vi "Write Control.vi"(6 "Data":u8[](array[numeric]), 8 "Error In":errorcluster, 9 "Device State":u32 format="%.0x", 10 "ADS State":T4, 11 "AMS Connection In":T1) -> (0 "Error Out":errorcluster, 2 "ADS Error":T3 items=["NoError"=0, "InternalError"=1, "NoRTime"=2, "LockedMemoryError"=3, "MailBoxError"=4, "WrongHMsg"=5, "TargetPortNotFound"=6, "TargetMachineNotFound"=7, "UnknownCommandID"=8, "BadTaskID"=9, "NoIO"=10, "UnknownAmsCommand"=11, "Win32Error"=12, "PortNotConnected"=13, "InvalidAmsLength"=14, "InvalidAmsNetID"=15, "AmsSyncAmsError"=22, "AmsSyncNoIndexMap"=23, "InvalidAmsPort"=24, "NoMemory"=25, "TCPSendError"=26, "HostUnreachable"=27, "NoLockedMemory"=1280, "MailboxFull"=1282, "DeviceError"=1792, "DeviceServiceNotSupported"=1793, "DeviceInvalidGroup"=1794, "DeviceInvalidOffset"=1795, "DeviceInvalidAccess"=1796, "DeviceInvalidSize"=1797, "DeviceInvalidData"=1798, "DeviceNotReady"=1799, "DeviceBusy"=1800, "DeviceInvalidContext"=1801, "DeviceNoMemory"=1802, "DeviceInvalidParam"=1803, "DeviceNotFound"=1804, "DeviceSyntaxError"=1805, "DeviceIncompatible"=1806, "DeviceExists"=1807, "DeviceSymboldNotFound"=1808, "DeviceSymbolVersionInvalid"=1809, "DeviceInvalidState"=1810, "DeviceTransModeNotSupported"=1811, "DeviceNotifyHandleInvalid"=1812, "DeviceClientUnknown"=1813, "DeviceNoMoreHandles"=1814, "DeviceInvalidWatchsize"=1815, "DeviceNotInitialized"=1816, "DeviceTimeOut"=1817, "DeviceNoInterface"=1818, "DeviceInvalidInterface"=1819, "DeviceInvalidCLSID"=1820, "DeviceInvalidObjectID"=1821, "ClientError"=1856, "ClientInvalidParameter"=1857, "ClientListEmpty"=1858, "ClientVariableInUse"=1859, "ClientDuplicateInvokeID"=1860, "ClientSyncTimeOut"=1861, "ClientW32OR"=1862, "ClientTimeoutInvalid"=1863, "ClientPortNotOpen"=1864, "ClientNoAmsAddr"=1865, "ClientSyncInternal"=1872, "ClientAddHash"=1873, "ClientRemoveHash"=1874, "ClientNoMoreSymbols"=1875, "ClientSyncResInvalid"=1876, "ClientSyncPortLocked"=1877, "ClientQueueFull"=1878], 3 "AMS Connection Out":T1)   [LabVIEW 2016, in "TwinCAT ADS.lvlib"]
uses:
  TwinCAT ADS.lvlib
  Low Level/TypeDefs/ADS States.ctl
  Low Level/TypeDefs/ADS Error.ctl
  Low Level/TypeDefs/AMS Connection.ctl
  Low Level/TypeDefs/AMS.ctl
  Low Level/TypeDefs/Command Id.ctl
  Low Level/TypeDefs/State Flag.ctl
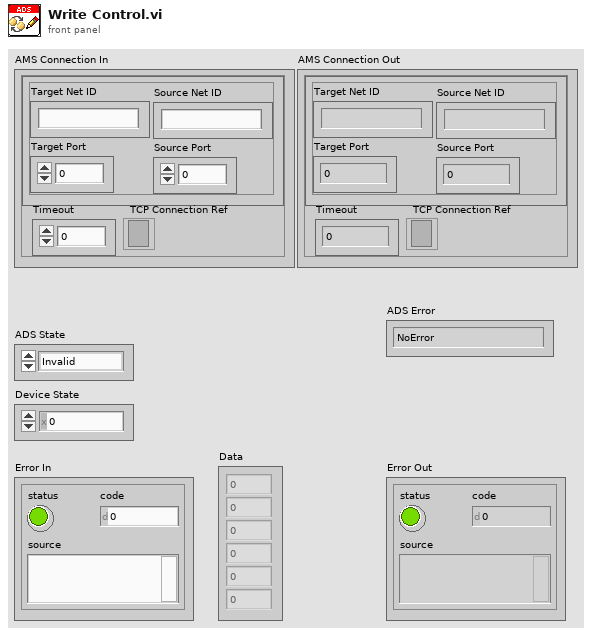
[diagram p1: front panel]
types:
  T1 = typedef "TwinCAT ADS.lvlib/AMS Connection.ctl" = cluster{"AMS":T2, "Timeout":i32, "TCP Connection Ref":refnum<k5>}
  T2 = typedef "TwinCAT ADS.lvlib/AMS.ctl" = cluster{"Target Net ID":string, "Target Port":u16, "Source Net ID":string, "Source Port":u16}
  T3 = typedef "TwinCAT ADS.lvlib/ADS Error.ctl" = i32
  T4 = typedef "TwinCAT ADS.lvlib/ADS States.ctl" = enum16{"Invalid", "Idle", "Reset", "Init", "Start", "Run", "Stop", "SaveCfg", "LoadCfg", "PowerFailure", "PowerGood", "Error", "Shutdown", "Suspend", "Resume", "Config", "Reconfig"}
  T5 = enum16{"Standard", "Buffered", "CRLF", "Immediate"}
  T6 = typedef "TwinCAT ADS.lvlib/State Flag.ctl" = u16
  T7 = typedef "TwinCAT ADS.lvlib/Command Id.ctl" = enum16{"Invalid", "ADS Read Device Info", "ADS Read", "ADS Write", "ADS Read State", "ADS Write Control", "ADS Add Device Notification", "ADS Delete Device Notification", "ADS Device Notification", "ADS Read Write"}
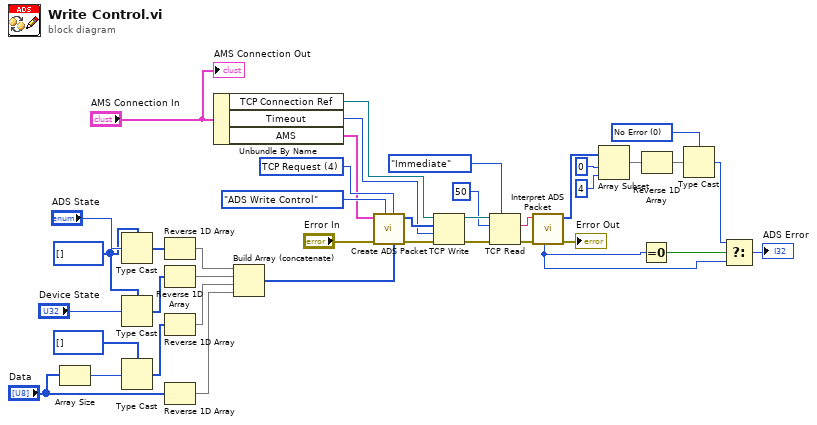
[diagram p0: block diagram]
diagram:
  w20 = T3 0 items=["No Error"] ("Enum")
  w8 = u8[] [] ("bytes to read")
  w39 = T6 4 items=["TCP Request"=4, "TCP Response"=5, "UDP Request"=68, "UDP Respone"=69] ("State Flag")
  n1 = Array Size(array="Data") -> (size(s)=w6:i32)
  n2 = Type Cast(type=w8, x="ADS State") -> (*(type *) &x=w27:u8[])
  n3 = Type Cast(type=w8, x="Device State") -> (*(type *) &x=w26:u8[])
  n4 = Type Cast(type=u8[] [] ("bytes to read"), x=w6) -> (*(type *) &x=w25:u8[])
  n5 = Reverse 1D Array(array=w27) -> (reversed array=w17:u8[])
  n6 = Reverse 1D Array(array=w26) -> (reversed array=w16:u8[])
  n7 = Reverse 1D Array(array=w25) -> (reversed array=w15:u8[])
  n8 = Reverse 1D Array(array="Data") -> (reversed array=w9:u8[])
  n9 = Unbundle By Name("AMS Connection In") -> ("TCP Connection Ref"=w3:refnum<k5>, "Timeout"=w2:i32, "AMS"=w4:T2)
  n10 = Build Array (concatenate)(w17, w16, w15, w9) -> (w24:u8[])
  n11 = call "Create ADS Packet.vi"("Data"=w24, "State Flag"=w39, "Command ID"=Command_Id."ADS Write Control", "Error In"="Error In", "AMS"=w4) -> ("Error Out"=w36:errorcluster, "ADS Packet"=w38:u8[])  [unwired: 5 in]
  n12 = TCP Write(connection ID=w3, data in=w38, error in (no error)=w36, 9:w2) -> (connection ID out=w37:refnum<k5>, error out=w35:errorcluster)  [unwired: 1 out]
  n13 = TCP Read(connection ID=w37, bytes to read=u32 50, error in (no error)=w35, 7:T5."Immediate" ("mode (standard)")) -> (data out=w31:string, error out=w32:errorcluster)  [unwired: 1 in, 1 out]
  n14 = call "Interpret ADS Packet.vi"("Error In"=w32, "ADS Packet"=w31) -> ("Error Out"=→"Error Out":errorcluster, "Data"=w19:u8[], "ADS Error"=w11:T3)  [unwired: 3 in, 4 out]
  n15 = Array Subset(array=w19, index=0, length=4) -> (w21:u8[])
  n16 = Equal To 0?(x=w11) -> (x = 0?=w13:bool)
  n17 = Reverse 1D Array(array=w21) -> (reversed array=w14:u8[])
  n18 = Type Cast(type=w20, x=w14) -> (*(type *) &x=w12:T3)
  n19 = Select(t=w12, s=w13, f=w11) -> (s? t:f=→"ADS Error":T3)
  "AMS Connection Out" <- "AMS Connection In"
